vi "Basic Set Pressure.vi"() -> ()   [LabVIEW 2016]
doc: "Purpose: This example shows how to set a pressure order and generate a triangle on the first pressure module of the chain \nHardware setup: At least one Fluigent pressure controller (MFCS, MFCS-EZ or FlowEZ)"
uses:
  fgt_SDK.lvlib
  <vilib>/ptbypt/NI_PtbyPt.lvlib
panel:
  in  "Stop button":bool
  out "error out":errorcluster
  out "Pressure chart":cluster{dbl, "pressure out":sgl}(graph)
  # "Hit the \"Run\" button to generate a pressure triangle"
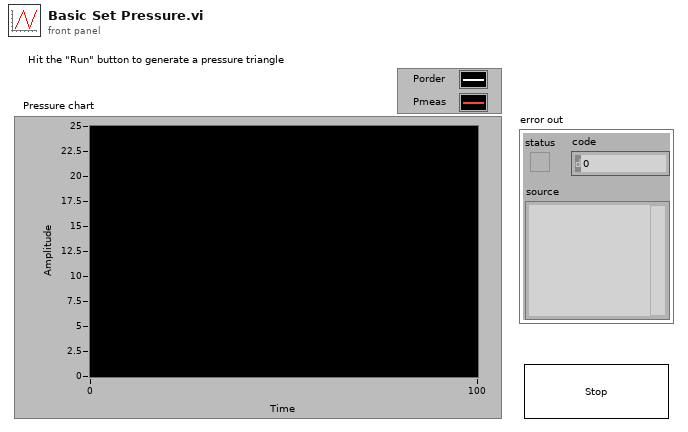
[diagram p1: front panel]
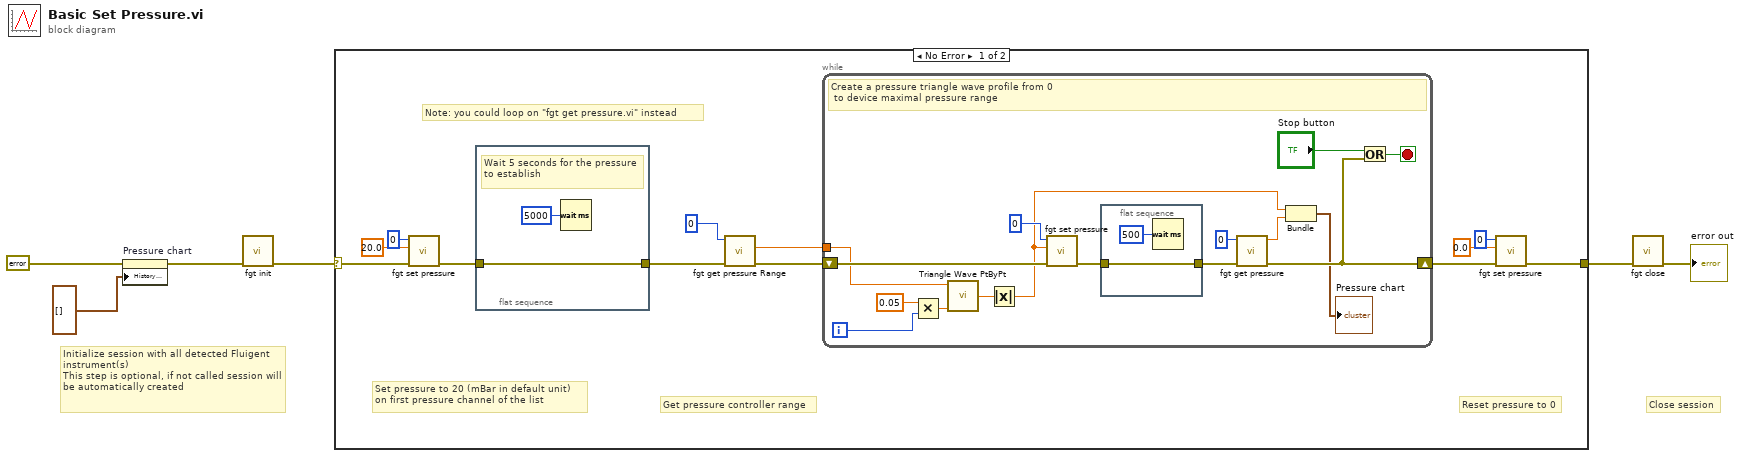
[diagram p0: block diagram]
diagram:
  # "Close session"
  # "Initialize session with all detected Fluigent instrument(s)\nThis step is optional, if not called session will be automatically created"
  n1 = property on="Pressure chart" class="WFChart (strict)"(error in=errorcluster {"status"=FALSE, "code"=0, "source"=""} ("error in (no error)"), "History Data"=cluster{dbl, "pressure out":sgl}[] []) -> (error out=w1:errorcluster)  [unwired: 1 in, 1 out]
  n2 = call "fgt init.vi"("error in (no error)"=w1) -> ("error out"=w3:errorcluster)  [unwired: 10 in]
  n3 = case shown="No Error" w3 {
    selector: w3 -> [w16 w39]
    tunnel: [w8 w39] -> w6
    frame No Error {
      # "Reset pressure to 0"
      # "Get pressure controller range"
      # "Set pressure to 20 (mBar in default unit) \non first pressure channel of the list"
      # "Note: you could loop on \"fgt get pressure.vi\" instead"
      n4 = call "fgt set pressure.vi"("error in (no error)"=w16, "pressure"=sgl 20.0, "pressureIndex"=u32 0) -> ("error out"=w15:errorcluster)  [unwired: 8 in]
      n5 = flat-sequence {
        tunnel: w15 -> [w37]
        tunnel: [w37] -> w14
        frame #0 {
          # "Wait 5 seconds for the pressure to establish"
          n6 = Wait (ms)(milliseconds to wait=u32 5000) -> ()  [unwired: 1 out]
        }
      }
      n7 = call "fgt get pressure Range.vi"("error in (no error)"=w14, "pressureIndex"=u32 0) -> ("error out"=w13:errorcluster, "Pmax out"=w7:sgl)  [unwired: 7 in, 1 out]
      n8 = while {
        shift-right: [w29] -> w10
        shift-left: w13 -> [w34]
        tunnel: w7 -> [w24]
        i -> [w26]
        stop <- w20 stop-if-true
        # "Create a pressure triangle wave profile from 0\n to device maximal pressure range"
        n9 = Multiply(x=0.05 ("time"), y=w26) -> (x*y=w27:dbl)
        n10 = call <vilib>:"Triangle Wave PtByPt.vi"("time"=w27, "amplitude"=w24) -> ("triangle wave"=w23:dbl)  [unwired: 2 in]
        n11 = Absolute Value(x=w23) -> (abs(x)=w22:dbl)
        n12 = call "fgt set pressure.vi"("error in (no error)"=w34, "pressure"=w22, "pressureIndex"=u32 0) -> ("error out"=w32:errorcluster)  [unwired: 8 in]
        n13 = flat-sequence {
          tunnel: [w35] -> w31
          tunnel: w32 -> [w35]
          frame #0 {
            n14 = Wait (ms)(milliseconds to wait=u32 500) -> ()  [unwired: 1 out]
          }
        }
        n15 = call "fgt get pressure.vi"("error in (no error)"=w31, "pressureIndex"=u32 0) -> ("error out"=w29:errorcluster, "pressure out"=w28:sgl)  [unwired: 8 in]
        n16 = Bundle(w22, "pressure out"=w28) -> (→"Pressure chart":cluster{dbl, "pressure out":sgl})  [unwired: 1 in]
        n17 = Or(x="Stop button", y=w29) -> (x .or. y?=w20:bool)
      }
      n18 = call "fgt set pressure.vi"("error in (no error)"=w10, "pressure"=sgl 0.0, "pressureIndex"=u32 0) -> ("error out"=w8:errorcluster)  [unwired: 8 in]
    }
    frame Error {
    }
  }
  n19 = call "fgt close.vi"("error in (no error)"=w6) -> ("error out"=→"error out":errorcluster)  [unwired: 10 in]
